vi "Test Get Progress when Running Filtered suite.vi"(8 "error in (no error)":errorcluster, 11 "Result Model Tests in":refnum<class "Result Model Statistics.lvclass">) -> (0 "error out":errorcluster, 3 "Result Model Tests out":refnum<class "Result Model Statistics.lvclass">)   [LabVIEW 2020, in "Result Model Statistics.lvclass"]
uses:
  Result Model Statistics.lvclass
  Result Model Statistics.lvclass/Result Model Statistics.ctl
  206db1ee-aa99-40b9-8881-171f2a77c34b.vi
  source/User Interface/Result Model by Reference/Result Model by Reference.lvclass
  Test Doubles/Test Case Test Double Child/Light Test Case Double.lvclass
  Test Doubles/Light Test Case Double Copy/Light Test Case Double Copy.lvclass
  source/LUnit Test Suite.lvclass
  C:/git/astemes-lunit/source/Core/Runnable/Runnable.lvclass
panel:
  out "Progress [%]":dbl
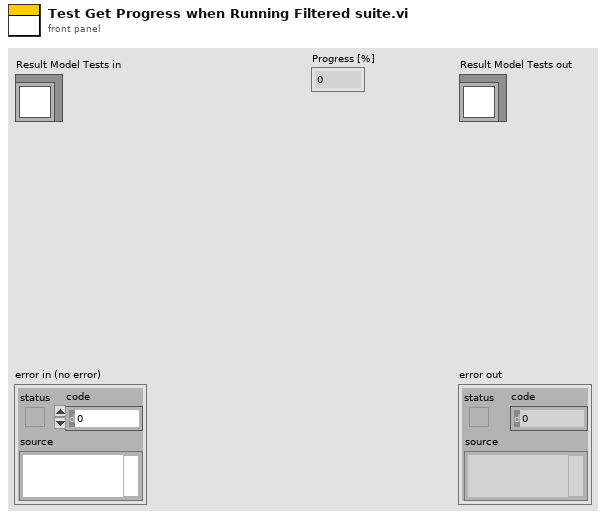
[diagram p1: front panel]
types:
  T1 = typedef "Result.lvlib/Result.ctl" = cluster{"Name":string, "Description":string, "Status":T2, "Result Type":T3, "Execution Time":dbl, "Data":cluster{"Expected":variant, "Actual":variant, "Delta":variant}}
  T2 = typedef "Result.lvlib/Status.ctl" = enum16{"", "Passed", "Failed", "Error", "Skipped", "Setup Error", "Broken", "Teardown Error"}
  T3 = typedef "Result.lvlib/Type.ctl" = enum16{"Test Case", "Test Suite", "Test Run", "Pass", "Fail", "Skip", "Pass if", "Fail if", "Pass if Error", "Fail if Error", "Pass if Equal", "Fail if Equal"}
  T4 = typedef "Result Model.lvclass/Statistics.ctl" = cluster{"Method Count":u32, "Executed Methods":u32, "Passed Methods":u32, "Failed Methods":u32, "Method Errors":u32, "Skipped Method":u32, "Progress [%]":dbl}
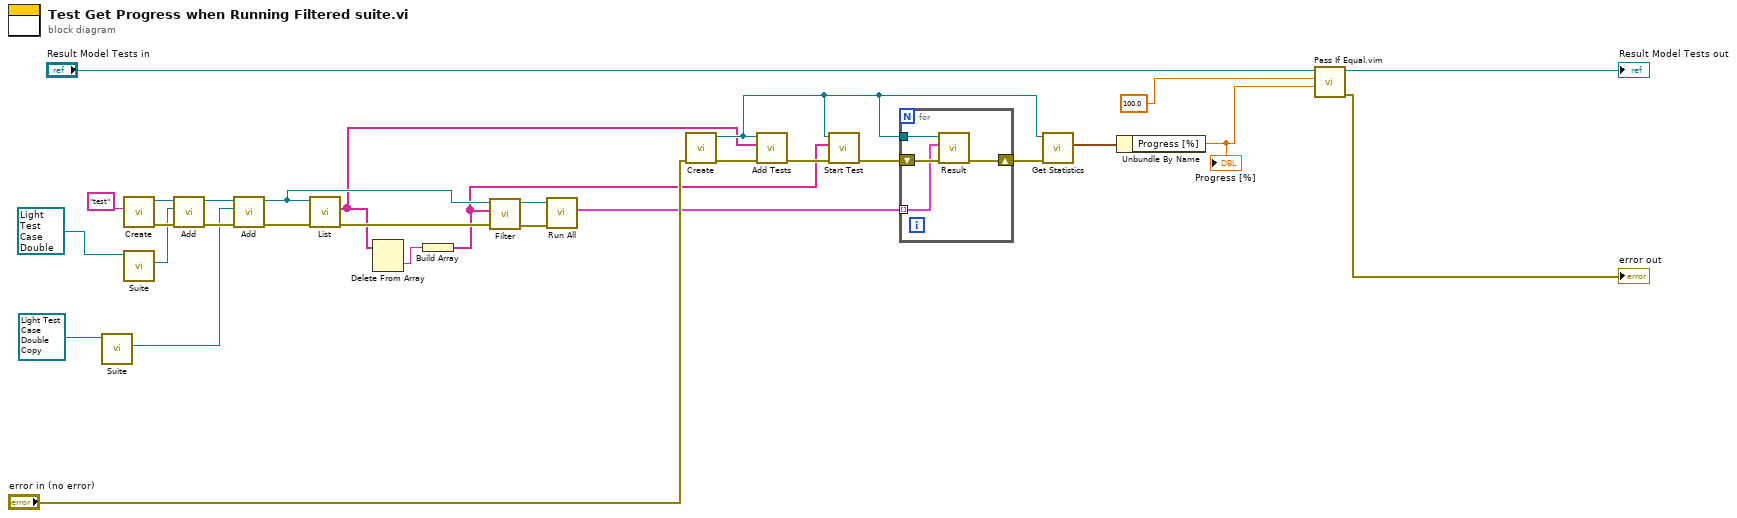
[diagram p0: block diagram]
diagram:
  n1 = call-dynamic "Suite.vi"("LUnit Test Case In"=refnum<class "Light Test Case Double Copy.lvclass"> refnum ("Light Test Case Double Copy.lvclass")) -> ("LUnit Test Suite Out"=w5:refnum<class "LUnit Test Suite.lvclass">)  [unwired: 8 in, 2 out]
  n2 = call "Create.vi"("Suite Name"="test") -> ("error out"=w10:errorcluster, "LUnit Test Suite Out"=w11:refnum<class "LUnit Test Suite.lvclass">)  [unwired: 9 in]
  n3 = call-dynamic "Suite.vi"("LUnit Test Case In"=refnum<class "Light Test Case Double.lvclass"> refnum ("Light Test Case Double.lvclass")) -> ("LUnit Test Suite Out"=w6:refnum<class "LUnit Test Suite.lvclass">)  [unwired: 8 in, 2 out]
  n4 = call "Add.vi"("error in (no error)"=w10, "Runnable"=w6, "LUnit Test Suite In"=w11) -> ("error out"=w8:errorcluster, "LUnit Test Suite Out"=w9:refnum<class "LUnit Test Suite.lvclass">)  [unwired: 7 in]
  n5 = call "Add.vi"("error in (no error)"=w8, "Runnable"=w5, "LUnit Test Suite In"=w9) -> ("error out"=w7:errorcluster, "LUnit Test Suite Out"=w4:refnum<class "LUnit Test Suite.lvclass">)  [unwired: 7 in]
  n6 = call "List.vi"("error in (no error)"=w7, "LUnit Test Suite In"=w4) -> ("error out"=w19:errorcluster, "List of Runnables"=w3:string[])  [unwired: 8 in]
  n7 = Delete From Array(array=w3) -> (deleted portion=w2:string)  [unwired: 2 in, 1 out]
  n8 = Build Array(w2) -> (w1:string[])
  n9 = call "Filter.vi"("error in (no error)"=w19, "Selected Runnables"=w1, "LUnit Test Suite In"=w4) -> ("error out"=w17:errorcluster, "LUnit Test Suite Out"=w18:refnum<class "LUnit Test Suite.lvclass">)  [unwired: 7 in]
  n10 = call "Run All.vi"("error in (no error)"=w17, "Runnable In"=w18) -> ("Results"=w16:T1[])  [unwired: 8 in, 1 out]
  n11 = call "Create.vi"("error in (no error)"="error in (no error)") -> ("error out"=w23:errorcluster, "Result Model out"=w14:refnum<class "Result Model by Reference.lvclass">)  [unwired: 9 in]
  n12 = call "Add Tests.vi"("error in (no error)"=w23, "Tests"=w3, "Result Model by Reference In"=w14) -> ("error out"=w15:errorcluster)  [unwired: 8 in]
  n13 = call "Start Test.vi"("error in (no error)"=w15, "Tests"=w1, "Result Model In"=w14) -> ("error out"=w22:errorcluster)  [unwired: 8 in]
  n14 = for {
    tunnel: w14 -> [w32]
    shift-right: [w33] -> w21
    shift-left: w22 -> [w34]
    tunnel: w16 -> [w31] mode=indexing
    n15 = call-dynamic "Result.vi"("error in (no error)"=w34, "Results"=w31, "Result Model by Reference In"=w32) -> ("error out"=w33:errorcluster)  [unwired: 8 in]
  }
  n16 = call "Get Statistics.vi"("error in (no error)"=w21, "Result Model in"=w14) -> ("Results"=w26:T4)  [unwired: 8 in, 1 out]
  n17 = Unbundle By Name(w26) -> ("Progress [%]"=w25:dbl)
  "Progress [%]" <- w25
  n18 = call "Pass If Equal.vim"("Actual"=w25, "Expected"=100.0 ("Method Count"), "LUnit Test Case In"="Result Model Tests in") -> ("error out"=→"error out":errorcluster, "LUnit Test Case Out"=→"Result Model Tests out":refnum<class "Result Model Statistics.lvclass">)  [unwired: 7 in]
